vi "JoystickRefNums.vi"() -> (0 "JoystickRefNums":T1)   [LabVIEW 2019]
uses:
  <vilib>/Rock Robotics/WPI/Joystick/WPI_JoystickDeviceEnum.ctl
  <vilib>/Rock Robotics/WPI/Joystick/WPI_JoystickDevRef.ctl
  TypeDefs/RobotComponents/JoystickRefNums.ctl
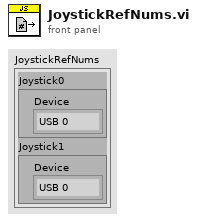
[diagram p1: front panel]
types:
  T1 = typedef "JoystickRefNums.ctl" = cluster{"Joystick0":T2, "Joystick1":T2}
  T2 = typedef "WPI_JoystickDevRef.ctl" = cluster{"Device":T3}
  T3 = typedef "WPI_JoystickDeviceEnum.ctl" = enum16{"USB 0", "USB 1", "USB 2", "USB 3", "USB 4", "USB 5"}
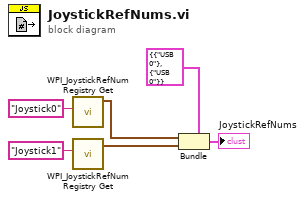
[diagram p0: block diagram]
diagram:
  n1 = call <vilib>:"WPI_JoystickRefNum Registry Get.vi"("refnum name"="Joystick0") -> ("JoystickDevRef"=w4:T2)  [unwired: 9 in, 1 out]
  n2 = call <vilib>:"WPI_JoystickRefNum Registry Get.vi"("refnum name"="Joystick1") -> ("JoystickDevRef"=w3:T2)  [unwired: 9 in, 1 out]
  n3 = Bundle(cluster=T1 {"Joystick0"={"Device"=enum."USB 0"}, "Joystick1"={"Device"=enum."USB 0"}} ("JoystickRefNums"), "Joystick0"=w4, "Joystick1"=w3) -> (→"JoystickRefNums":T1)
